vi "Aktualizacja listy z punktami + startem.vi"(10 "Lista współrzędnych":string[][](array[string]), 11 "Lista z punktami do usunięcia":refnum<vi>) -> ()   [LabVIEW 2012, in "Biblioteka moduł map v3.lvlib" / "Obsługa listy współrzędnych.lvlib"]
doc: "Dodanie do kontrolki enumerate nazw wszystkich punktów znajdujących sie na liście współrzędnych."
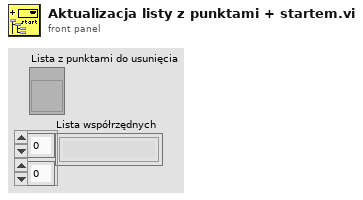
[diagram p1: front panel]
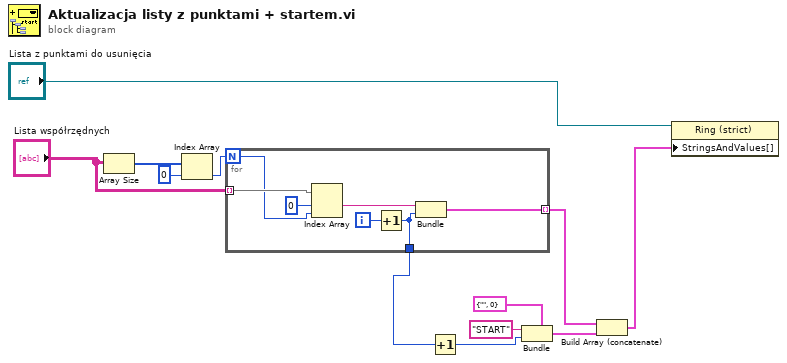
[diagram p0: block diagram]
diagram:
  n1 = Array Size(array="Lista współrzędnych") -> (size(s)=w10:i32[])
  n2 = Index Array(array=w10, index=0) -> (element=w8:i32)
  n3 = for {
    N: w8 -> [w15]
    tunnel: "Lista współrzędnych" -> [w19] mode=indexing
    tunnel: [w17] -> w2 mode=indexing
    tunnel: [w13] -> w3
    i -> [w16]
    n4 = Index Array(array=w19, index #1=0 ("index"), index #2=w15) -> (element #1=w18:string)  [unwired: 1 out]
    n5 = Increment(x=w16) -> (x+1=w13:i32)
    n6 = Bundle(w18, w13) -> (w17:cluster{string, i32})  [unwired: 1 in]
  }
  n7 = Increment(x=w3) -> (x+1=w5:i32)
  n8 = Bundle(cluster=cluster{string, i32} {"", 0}, "START", w5) -> (w4:cluster{string, i32})
  n9 = Build Array (concatenate)(w2, w4) -> (w1:cluster{string, i32}[])
  n10 = property class="Ring (strict)"(reference="Lista z punktami do usunięcia", "StringsAndValues[]"=w1) -> ()  [unwired: 1 in, 2 out]
